vi "Transform2d_GetTranslation.vi"(11 "inTRANSFORM":T2={"TRANSLATION"={"X"=0.0, "Y"=0.0}, "ROTATION"={"VALUE"=0.0, "COS"=1.0, "SIN"=0.0}, "xF"=FALSE} {"ROTATION"."SIN" format="%13.4f"; "ROTATION"."COS" format="%13.4f"; "ROTATION"."VALUE" format="%13.4f"; "TRANSLATION"."Y" format="%14.3f"; "TRANSLATION"."X" format="%14.3f"}) -> (3 "TRANSLATION":T1 {"Y" format="%14.3f"; "X" format="%14.3f"})   [LabVIEW 2019, in "Trajectory_Library.lvlib"]
doc: "Returns the translation component of the transformation.\n\nParameters:\n - IN TRANSFORM - THis TRANSFORM data structure\n\nReturns:\n - TRANSLATION - The translational component of the transform."
uses:
  Trajectory_Library.lvlib
  TypeDef/TRANSFORM2D.ctl
  TypeDef/TRANSLATION2D.ctl
  TypeDef/ROTATION2D.ctl
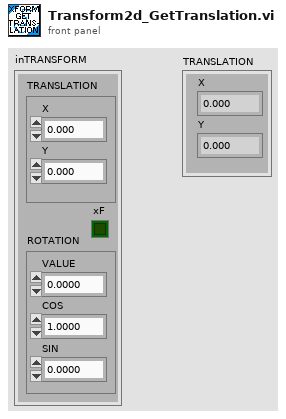
[diagram p1: front panel]
types:
  T1 = typedef "Trajectory_Library.lvlib/TRANSLATION2D.ctl" = cluster{"X":dbl, "Y":dbl}
  T2 = typedef "Trajectory_Library.lvlib/TRANSFORM2D.ctl" = cluster{"TRANSLATION":T1, "ROTATION":T3, "xF":bool}
  T3 = typedef "Trajectory_Library.lvlib/ROTATION2D.ctl" = cluster{"VALUE":dbl, "COS":dbl, "SIN":dbl}
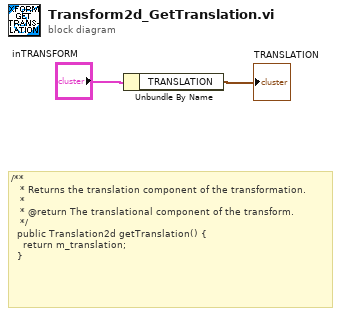
[diagram p0: block diagram]
diagram:
  # "/**\n   * Returns the translation component of the transformation.\n   *\n   * @return The translational component of the transform.\n   */\n  public Translation2d getTranslation() {\n    return m_translation;\n  }"
  n1 = Unbundle By Name("inTRANSFORM") -> ("TRANSLATION"=→"TRANSLATION":T1)
